vi "Write inter-frame delay.vi"(8 "error in (no error)":errorcluster, 10 "inter-frame delay":u32=2, 11 "MB_ADU_Serial_RTU in":refnum<class "MB_ADU_RTU.lvclass">) -> (0 "error out":errorcluster, 3 "MB_ADU_Serial_RTU out":refnum<class "MB_ADU_RTU.lvclass">)   [LabVIEW 2012, in "MB Master.lvlib" / "MB_ADU_RTU.lvclass"]
uses:
  MB_ADU_RTU.lvclass
  MB_ADU_RTU.lvclass/MB_ADU_RTU.ctl
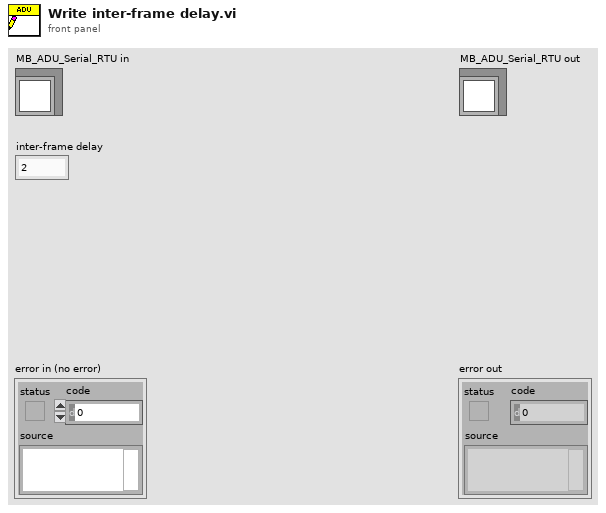
[diagram p1: front panel]
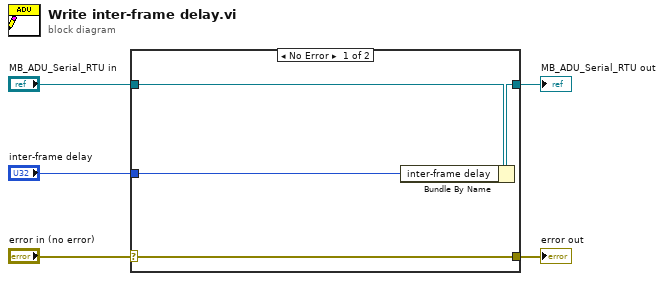
[diagram p0: block diagram]
diagram:
  n1 = case shown="No Error" "error in (no error)" {
    selector: "error in (no error)" -> [w9 w10]
    tunnel: [w9 w10] -> w4
    tunnel: [w7 w11] -> w2
    tunnel: "MB_ADU_Serial_RTU in" -> [w8 w11]
    tunnel: "inter-frame delay" -> [w6 _]
    frame No Error {
      n2 = Bundle By Name(cluster=w8, "inter-frame delay"=w6) -> (w7:refnum<class "MB_ADU_RTU.lvclass">)
    }
    frame Error {
    }
  }
  "error out" <- w4
  "MB_ADU_Serial_RTU out" <- w2
